vi "Voice Level Controls.vi"(8 "error in":errorcluster, 11 "MIDI Controls in":T2=variant(dbl 0.0)) -> (0 "error out":errorcluster, 2 "Voice Level Controls out":T1)   [LabVIEW 2014, in "mySynthesizer.lvlib" / "Voice Level Controls.lvlib"]
uses:
  Voice Level Controls.lvlib
  MIDI Controls/MIDI Controls.ctl
  Voice Level Controls.ctl
  MIDI Controls/MIDI Controls.lvlib
panel:
  in  "error in (no error)":errorcluster
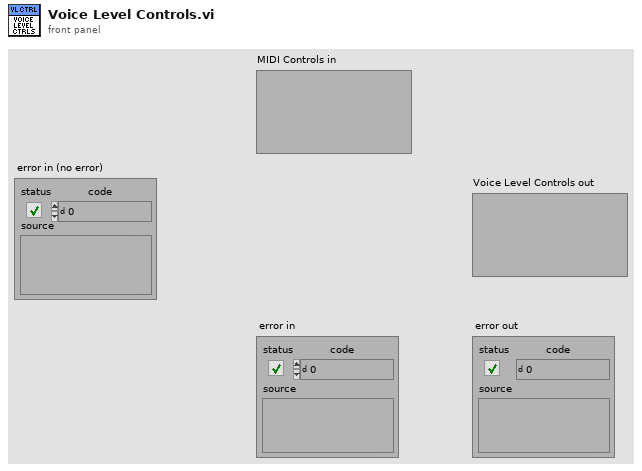
[diagram p1: front panel]
types:
  T1 = typedef "mySynthesizer.lvlib/Voice Level Controls.lvlib/Voice Level Controls.ctl" = variant
  T2 = typedef "mySynthesizer.lvlib/MIDI Controls.lvlib/MIDI Controls.ctl" = variant
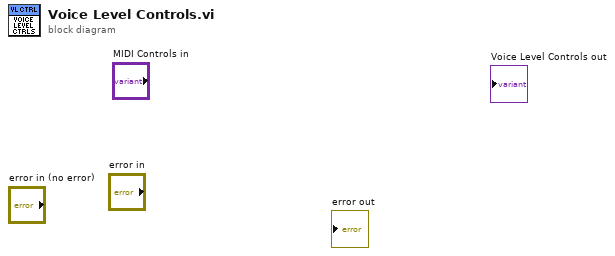
[diagram p0: block diagram]
diagram:
